vi "Count Coins - Image.vi"() -> ()   [LabVIEW 2023]
uses:
  Coin Analyser/Coins.ctl
  Coin Analyser/Coin Analyser.lvclass
panel:
  out "Features":cluster{"x":i32, "y":i32, "diameter":i32}[](array[cluster])
  out "Image":T1(plugin-control)
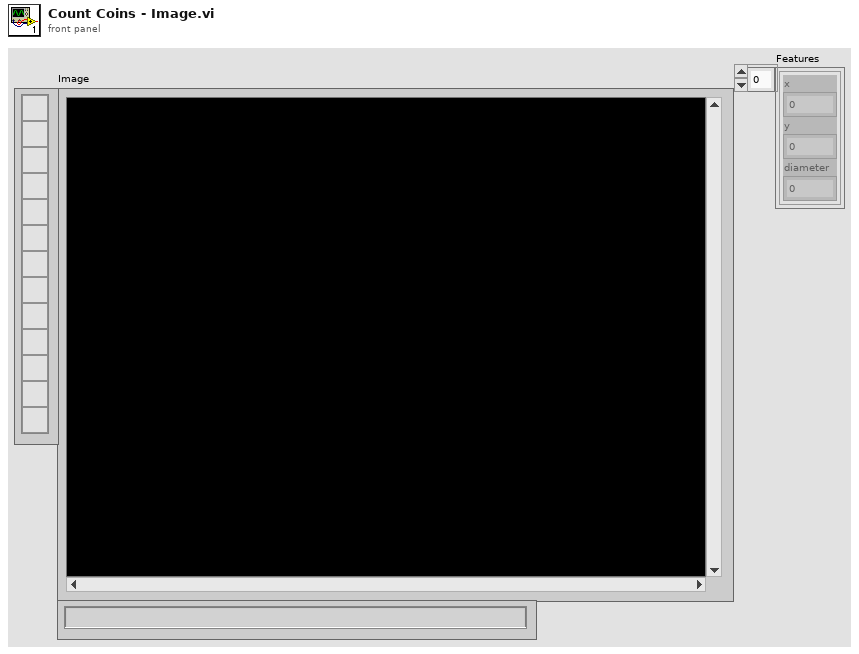
[diagram p1: front panel]
types:
  T1 = typedef "IMAQ Image.ctl" = refnum<image>
  T2 = typedef "Coin Analyser.lvclass/Coins.ctl" = cluster{"x":i32, "y":i32, "diameter":i32}
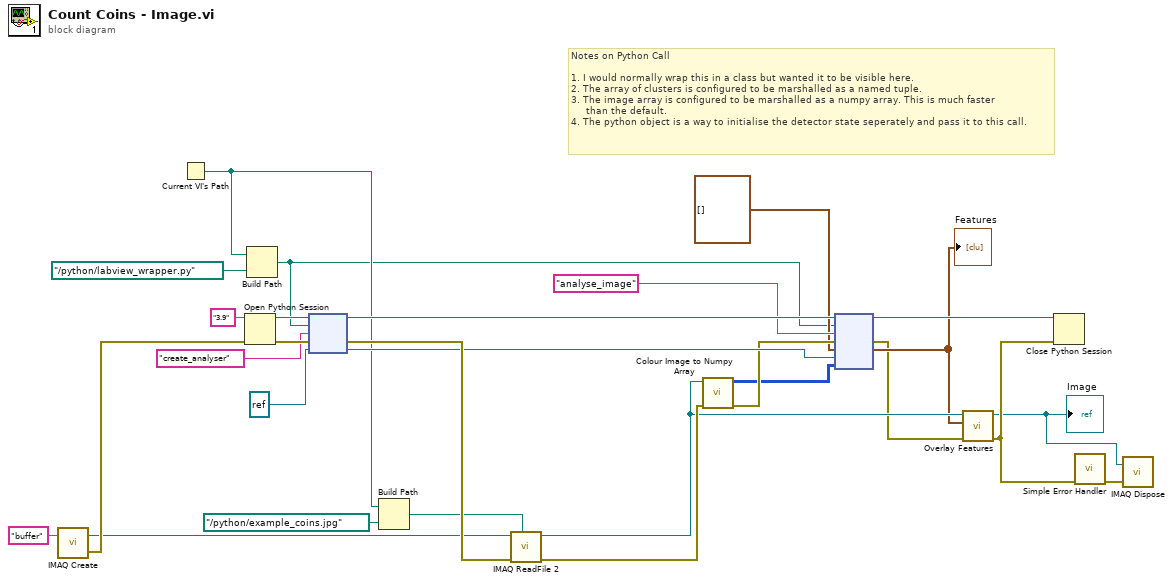
[diagram p0: block diagram]
diagram:
  # "Notes on Python Call\n\n1. I would normally wrap this in a class but wanted it to be visible here.\n2. The array of clusters is configured to be marshalled as a named tuple.\n3. The image array is configured to be marshalled as a numpy array. This is much faster\n     than the default.\n4. The python object is a way to initialise the detector state seperately and pass it to this call."
  n1 = call "IMAQ Create"("Image Name"="buffer") -> ("New Image"=w16:T1, "error out"=w17:errorcluster)  [unwired: 4 in]
  n2 = Current VI's Path() -> (path=w2:path)
  n3 = Open Python Session(python version="3.9" ("Python version"), 3:w17) -> (session out=w26:refnum<k35>, error out=w25:errorcluster)  [unwired: 1 in]
  n4 = Build Path(base path=w2, name or relative path=path "../python/labview_wrapper.py" ("module path")) -> (appended path=w1:path)
  n5 = node(w26, w1, "create_analyser" ("function name"), w25, refnum<k38> refnum ("Python Object Refnum")) -> (w22:refnum<k35>, w24:errorcluster, w20:refnum<k38>)  [unwired: 2 out]
  n6 = Build Path(base path=w2, name or relative path=path "../python/example_coins.jpg") -> (appended path=w6:path)
  n7 = call "IMAQ ReadFile 2"("File Path"=w6, "error in (no error)"=w24, "Image"=w16) -> ("error out"=w19:errorcluster, "Image Out"=w15:T1)  [unwired: 4 in, 3 out]
  n8 = call "Colour Image to Numpy Array.vi"("error in (no error)"=w19, "Refnum in"=w15) -> ("error out"=w12:errorcluster, "Array"=w9:u8[][][])  [unwired: 8 in]
  n9 = node(w22, w1, "analyse_image" ("function name"), w12, T2[] [], w20, w9) -> (w21:refnum<k35>, w8:errorcluster, w10:T2[])  [unwired: 2 in, 2 out]
  "Features" <- w10
  n10 = call "Overlay Features.vi"("error in (no error)"=w8, "Features"=w10, "Refnum in"=w15) -> ("Error Out"=w14:errorcluster, "Refnum out"=w4:T1)  [unwired: 7 in]
  "Image" <- w4
  n11 = Close Python Session(session in=w21, error in=w14) -> ()  [unwired: 1 out]
  n12 = call <vilib>:"Simple Error Handler.vi"("error in (no error)"=w14) -> ("error out"=w5:errorcluster)  [unwired: 4 in, 4 out]
  n13 = call "IMAQ Dispose"("Image"=w4, "error in (no error)"=w5) -> ()  [unwired: 4 in, 1 out]
